vi "teleop_v4.vi"() -> ()   [LabVIEW 2012, in "MainProject.lvrbt"]
uses:
  MainProject.lvrbt
  <vilib>/NXT/Hardware/Plugins/Tetrix 180 deg Servo/Tetrix180ServoAddress.ctl
  <vilib>/NXT/Hardware/Plugins/Tetrix DC Motor/TetrixDCMotorAddress.ctl
  <vilib>/NXT/HiTechnic/HiTechnic Controls/HiTechnic Port.ctl
  <vilib>/NXT/Block Support/NXT_InputPort.ctl
  <vilib>/NXT/Hardware/Plugins/Tetrix Continuous Servo/TetrixContinuousServoAddress.ctl
  Drivers/AutoDriverControl.ctl
  <vilib>/NXT/Dual Mode Library/Advanced/NXTFlag_Get_Integer.vi
  <vilib>/NXT/NXTIO Xnodes/NXTIONodeSubVIs/TETRIX IO Stop DC Motors.vi
  <vilib>/NXT/NXTIO Xnodes/NXTIONodeSubVIs/TETRIX IO Move DC Motors.vi
  <vilib>/NXT/Dual Mode Library/Sound/Tone.vi
  <vilib>/NXT/NXTIO Xnodes/NXTIONodeSubVIs/TETRIX IO Move Servos.vi
  <vilib>/NXT/Dual Mode Library/Advanced/NXTFlag_Assign_integer.vi
  <vilib>/NXT/NXTIO Xnodes/NXTIONodeSubVIs/TETRIX IO Move Continuous Servos.vi
  <vilib>/NXT/NXTIO Xnodes/NXTIONodeSubVIs/TETRIX IO Stop Continuous Servos.vi
  <vilib>/FTC/FTC Calculate Drive Power - Tank.vi
  <vilib>/NXT/NXTIO Xnodes/NXTIONodeSubVIs/TETRIX IO Check Battery.vi
  <vilib>/NXT/Subs/LVHSConnector.ctl
  <vilib>/NXT/NXTIO Xnodes/AddressXNode/NXTIOAddress.xnode
  <vilib>/NXT/NXTIO Xnodes/NXTIOXNode/NXTIO.xnode
  <vilib>/NXT/LegoClasses/BrickReference/BrickReference.lvclass
panel:
  out "Drive Power":i8=75 min=-100 max=100
  # "This VI was generated based on your configuration in the Remote Control Editor. You may modify the code as needed for your robot. To test this program for an FTC match, return to the Remote Control Editor, select the \"Run Program\" tab, and choose \"Teleop\"."
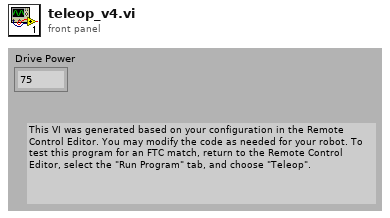
[diagram p1: front panel]
types:
  T1 = typedef "Tetrix180ServoAddress.ctl" = i16
  T2 = cluster{"Tetrix180Servo":T1, "Tetrix180Servo":T1, "Tetrix180Servo":T1}
  T3 = typedef "LVHSConnector.ctl" = refnum<class "BrickReference.lvclass">
  T4 = typedef "TetrixDCMotorAddress.ctl" = i16
  T5 = cluster{"TetrixDCMotor":T4, "TetrixDCMotor 2":T4}
  T6 = typedef "AutoDriverControl.ctl" = enum16{"Init", "Forward", "Reverse", "Left", "Right", "Brake"}
  T7 = typedef "FTC ControllerState.ctl" = cluster{"Left X":i8, "Left Y":i8, "Right X":i8, "Right Y":i8, "Button Encoding 9-12":u8, "Button Encoding 1-8":u8, "POV":T8}
  T8 = typedef "FTC POVState.ctl" = i8
  T9 = typedef "FTC ButtonEventType.ctl" = enum16{"Pressed", "Released"}
  T10 = cluster{"Button ID":enum16{"None", "Button 1", "Button 2", "Button 3", "Button 4", "Button 5", "Button 6", "Button 7", "Button 8", "Button 9", "Button 10", "Button 11", "Button 12", "POV Up", "POV Up Right", "POV Right", "POV Down Right", "POV Down", "POV Down Left", "POV Left", "POV Up Left"}, "Event Type":T9}[]
  T11 = enum16{"None", "Button 1", "Button 2", "Button 3", "Button 4", "Button 5", "Button 6", "Button 7", "Button 8", "Button 9", "Button 10", "Button 11", "Button 12", "POV Up", "POV Up Right", "POV Right", "POV Down Right", "POV Down", "POV Down Left", "POV Left", "POV Up Left"}
  T12 = typedef "TetrixContinuousServoAddress.ctl" = i16
  T13 = typedef "HiTechnic Port.ctl" = cluster{"Port":T14, "MUX Port":u8}
  T14 = typedef "NXT_InputPort.ctl" = u8
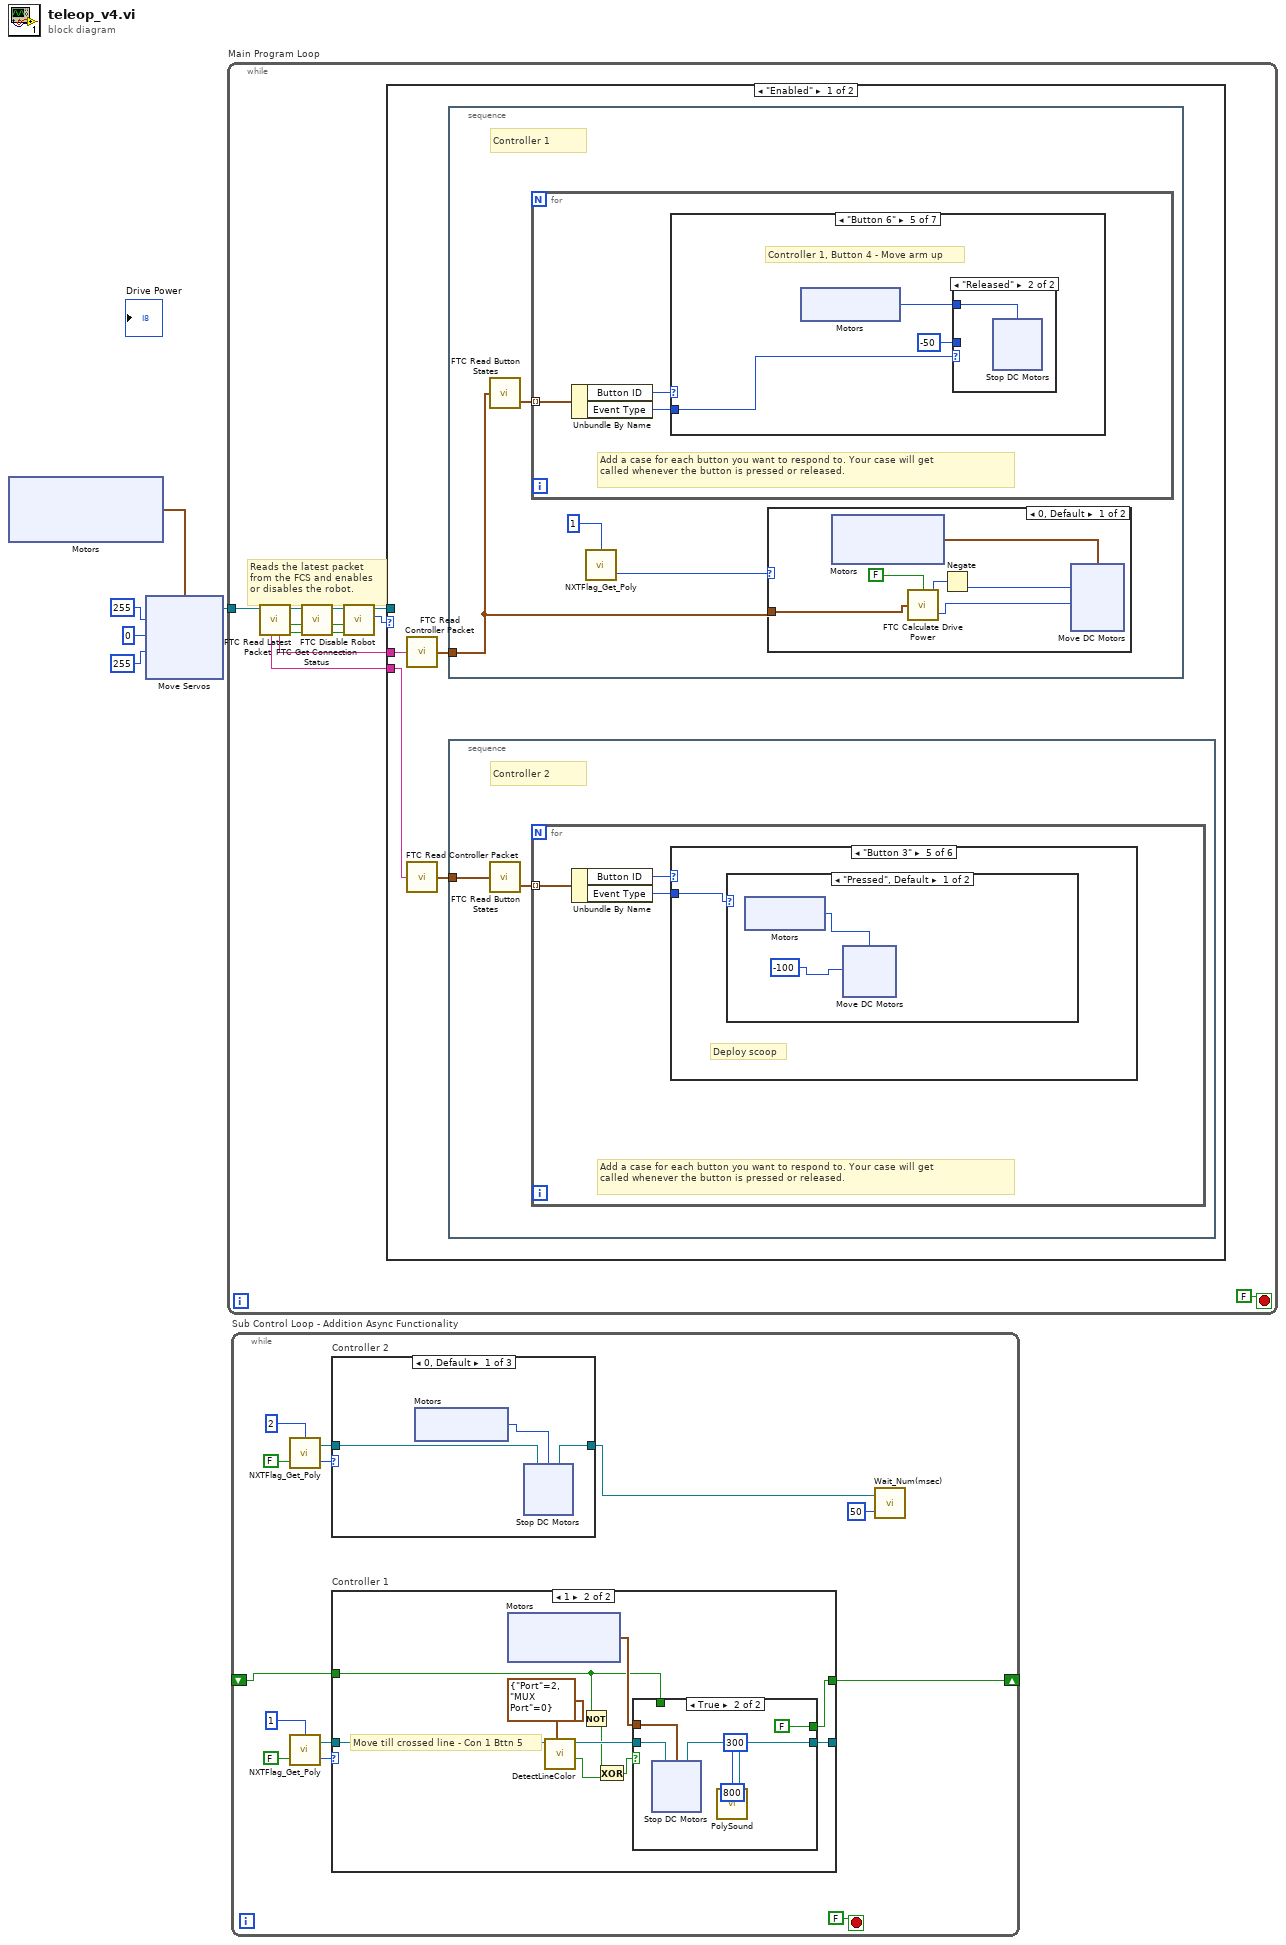
[diagram p0: block diagram]
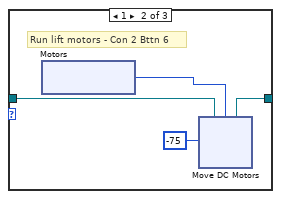
[diagram p2: hidden frame]
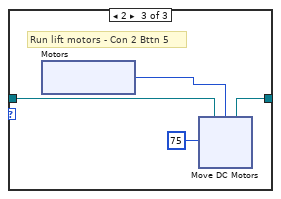
[diagram p3: hidden frame]
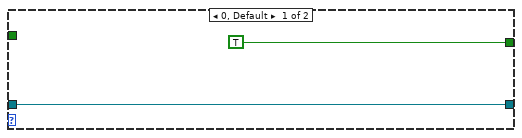
[diagram p4: hidden frame]
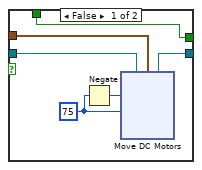
[diagram p5: hidden frame]
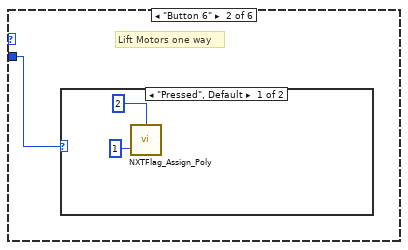
[diagram p7: hidden frame]
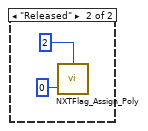
[diagram p8: hidden frame]
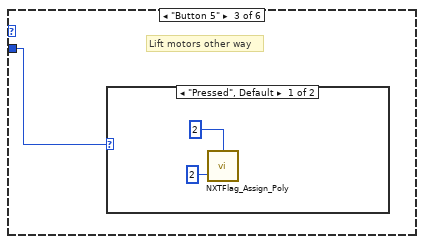
[diagram p9: hidden frame]
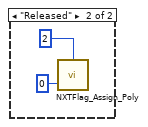
[diagram p10: hidden frame]
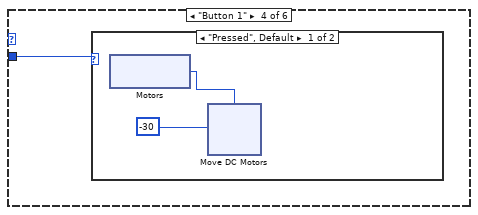
[diagram p11: hidden frame]
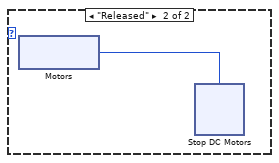
[diagram p12: hidden frame]
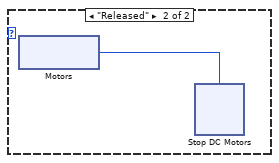
[diagram p13: hidden frame]
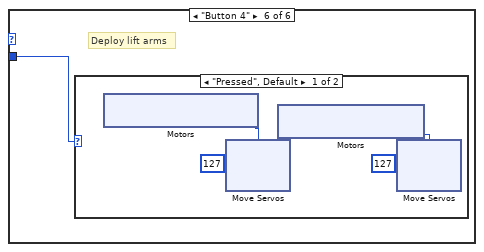
[diagram p14: hidden frame]
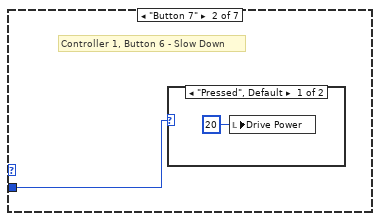
[diagram p18: hidden frame]
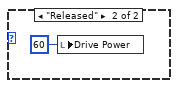
[diagram p19: hidden frame]
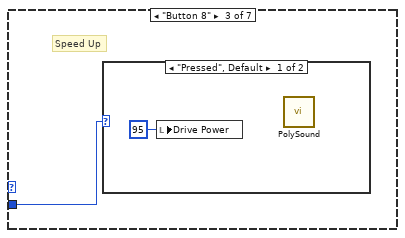
[diagram p20: hidden frame]
diagram:
  n1 = xnode "Motors"() -> ("Motor"=w4:T2)
  n2 = xnode "Move Servos"("Position 2"=u8 0, "Position 1"=u8 255, "Servos"=w4, "Position 3"=u8 255) -> ("NXT"=w5:T3)  [unwired: 1 in]
  n3 = while "Main Program Loop" {
    tunnel: w5 -> [w6]
    stop <- FALSE stop-if-true
    # "Reads the latest packet\nfrom the FCS and enables\nor disables the robot."
    n4 = call <vilib>:"FTC Read Latest Packet.vi"("NXT"=w6) -> ("Packet Received?"=w14:bool, "Stopped?"=w11:bool, "NXT"=w13:T3, "Controller 1"=w16:string, "Controller 2"=w15:string)  [unwired: 5 in, 1 out]
    n5 = call <vilib>:"FTC Get Connection Status.vi"("Packet Received?"=w14, "Stopped?"=w11, "NXT"=w13) -> ("Online?"=w8:bool, "Stopped?"=w9:bool, "NXT"=w10:T3)  [unwired: 5 in]
    n6 = call <vilib>:"FTC Disable Robot.vi"("Online?"=w8, "Stopped?"=w9, "NXT"=w10) -> ("Enabled?"=w12:enum16{"Disabled", "Enabled"}, "NXT"=w7:T3)  [unwired: 3 in]
    n7 = case "disableCase" shown="\"Enabled\"" w12 {
      tunnel: w16 -> [w21 _]
      tunnel: w15 -> [w20 _]
      tunnel: w7 -> [_ w207]
      frame "Enabled" {
        n8 = call <vilib>:"FTC Read Controller Packet.vi"("Packet"=w21) -> ("Controller State"=w19:T7)  [unwired: 4 in]
        n9 = call <vilib>:"FTC Read Controller Packet.vi"("Packet"=w20) -> ("Controller State"=w18:T7)  [unwired: 4 in]
        n10 = stacked-sequence "controller1Actions" {
          tunnel: w19 -> [w94]
          frame #0 {
            # "Controller 1"
            n11 = call <vilib>:"FTC Read Button States.vi"("Controller State"=w94) -> ("Button Events"=w97:T10)  [unwired: 2 in, 1 out]
            n12 = for "buttonAction" {
              tunnel: w97 -> [w115] mode=indexing
              # "Add a case for each button you want to respond to. Your case will get \ncalled whenever the button is pressed or released."
              n13 = Unbundle By Name(w115) -> ("Button ID"=w117:T11, "Event Type"=w116:T9)
              n14 = case "EventCase1" shown="\"Button 6\"" w117 {
                tunnel: w116 -> [_ w118 w121 w124 w134 w153 w174]
                frame Default {
                  # "No Action"
                }
                frame "Button 7" {
                  # "Controller 1, Button 6 - Slow Down"
                  n15 = case shown="\"Pressed\", Default" w118 {
                    frame "Pressed", Default {
                      n16 = local write "Drive Power"(i8 20 ("Drive Power")) -> ()
                    }
                    frame "Released" {
                      n17 = local write "Drive Power"(i8 60 ("Drive Power")) -> ()
                    }
                  }
                }
                frame "Button 8" {
                  # "Speed Up"
                  n18 = case shown="\"Pressed\", Default" w121 {
                    frame "Pressed", Default {
                      n19 = local write "Drive Power"(i8 95 ("Drive Power")) -> ()
                      n20 = call-poly <vilib>:"PolySound.vi"() -> ()  [unwired: 4 in, 1 out]
                    }
                    frame "Released" {
                      n21 = local write "Drive Power"(i8 60 ("Drive Power")) -> ()
                    }
                  }
                }
                frame "Button 2" {
                  # "Drive forward till hit line"
                  n22 = case shown="\"Released\"" w124 {
                    frame "Pressed", Default {
                      n23 = call-poly <vilib>:"NXTFlag_Assign_Poly.vi"("Flag Value"=1, "NXT Flag Number"=i8 1) -> ()  [unwired: 2 in, 1 out]
                    }
                    frame "Released" {
                      n24 = call-poly <vilib>:"NXTFlag_Assign_Poly.vi"("Flag Value"=0, "NXT Flag Number"=i8 1) -> ("NXT"=w128:T3)  [unwired: 2 in]
                      n25 = xnode "Motors"() -> ("Motor"=w130:cluster{"TetrixDCMotor":T4, "TetrixDCMotor":T4})
                      n26 = call "AutoDriver.vi"("NXT In"=w128, "Motors"=w130, "Direction"=AutoDriverControl."Brake", "Time (1 sec)"=sgl 0.0001) -> ()  [unwired: 4 in, 1 out]
                    }
                  }
                }
                frame "Button 6" {
                  # "Controller 1, Button 4 - Move arm up"
                  n27 = xnode "Motors"() -> ("Motor"=w135:T4)
                  n28 = case shown="\"Released\"" w134 {
                    tunnel: -50 ("Power (75)") -> [w139 _]
                    tunnel: w135 -> [w138 w147]
                    frame "Pressed", Default {
                      n29 = xnode "Move DC Motors"("Power/Speed 1"=w139, "Motors"=w138) -> ()  [unwired: 1 in, 1 out]
                    }
                    frame "Released" {
                      n30 = xnode "Stop DC Motors"("Motors"=w147) -> ()  [unwired: 1 in, 1 out]
                    }
                  }
                }
                frame "Button 1" {
                  # "Open Block Door Servo"
                  n31 = case shown="\"Pressed\", Default" w153 {
                    frame "Pressed", Default {
                      n32 = xnode "Motors"() -> ("Motor"=w155:T1)
                      n33 = xnode "Move Servos"("Position 1"=u8 10, "Servos"=w155) -> ()  [unwired: 1 in, 1 out]
                    }
                    frame "Released" {
                      n34 = xnode "Motors"() -> ("Motor"=w165:T1)
                      n35 = xnode "Move Servos"("Position 1"=u8 255, "Servos"=w165) -> ()  [unwired: 1 in, 1 out]
                    }
                  }
                }
                frame "Button 5" {
                  # "Controller 1, Button 2 - Move arm down"
                  n36 = xnode "Motors"() -> ("Motor"=w175:T4)
                  n37 = case shown="\"Pressed\", Default" w174 {
                    tunnel: 50 ("Power (75)") -> [w179 _]
                    tunnel: w175 -> [w178 w187]
                    frame "Pressed", Default {
                      n38 = xnode "Move DC Motors"("Power/Speed 1"=w179, "Motors"=w178) -> ()  [unwired: 1 in, 1 out]
                    }
                    frame "Released" {
                      n39 = xnode "Stop DC Motors"("Motors"=w187) -> ()  [unwired: 1 in, 1 out]
                    }
                  }
                }
              }
            }
            n40 = call-poly <vilib>:"NXTFlag_Get_Poly.vi"("NXT Flag Number"=1) -> ("Flag Value"=w95:i32)  [unwired: 2 in, 1 out]
            n41 = case shown="0, Default" w95 {
              tunnel: w94 -> [w98 _]
              frame 0, Default {
                n42 = xnode "Motors"() -> ("Motor"=w102:cluster{"TetrixDCMotor":T4, "TetrixDCMotor":T4})
                n43 = call-poly <vilib>:"FTC Calculate Drive Power.vi"("Reverse"=FALSE, "Controller State"=w98) -> ("Right Motor Power"=w100:i8, "Left Motor Power"=w101:i8)  [unwired: 2 in]
                n44 = Negate(x=w101) -> (-x=w99:i8)
                n45 = xnode "Move DC Motors"("Power/Speed 2"=w100, "Power/Speed 1"=w99, "Motors"=w102) -> ()  [unwired: 1 in, 1 out]
              }
              frame 1 {
              }
            }
          }
        }
        n46 = stacked-sequence "controller2Actions" {
          tunnel: w18 -> [w22]
          frame #0 {
            # "Controller 2"
            n47 = call <vilib>:"FTC Read Button States.vi"("Controller State"=w22) -> ("Button Events"=w23:T10)  [unwired: 2 in, 1 out]
            n48 = for "buttonAction" {
              tunnel: w23 -> [w24] mode=indexing
              # "Add a case for each button you want to respond to. Your case will get \ncalled whenever the button is pressed or released."
              n49 = Unbundle By Name(w24) -> ("Button ID"=w26:T11, "Event Type"=w25:T9)
              n50 = case "EventCase2" shown="\"Button 3\"" w26 {
                tunnel: w25 -> [_ w27 w32 w37 w55 w73]
                frame Default {
                  # "No Action"
                }
                frame "Button 6" {
                  # "Lift Motors one way"
                  n51 = case shown="\"Pressed\", Default" w27 {
                    frame "Pressed", Default {
                      n52 = call-poly <vilib>:"NXTFlag_Assign_Poly.vi"("Flag Value"=1, "NXT Flag Number"=i8 2) -> ()  [unwired: 2 in, 1 out]
                    }
                    frame "Released" {
                      n53 = call-poly <vilib>:"NXTFlag_Assign_Poly.vi"("Flag Value"=0, "NXT Flag Number"=i8 2) -> ()  [unwired: 2 in, 1 out]
                    }
                  }
                }
                frame "Button 5" {
                  # "Lift motors other way"
                  n54 = case shown="\"Pressed\", Default" w32 {
                    frame "Pressed", Default {
                      n55 = call-poly <vilib>:"NXTFlag_Assign_Poly.vi"("Flag Value"=2, "NXT Flag Number"=i8 2) -> ()  [unwired: 2 in, 1 out]
                    }
                    frame "Released" {
                      n56 = call-poly <vilib>:"NXTFlag_Assign_Poly.vi"("Flag Value"=0, "NXT Flag Number"=i8 2) -> ()  [unwired: 2 in, 1 out]
                    }
                  }
                }
                frame "Button 1" {
                  n57 = case shown="\"Pressed\", Default" w37 {
                    frame "Pressed", Default {
                      n58 = xnode "Motors"() -> ("Motor"=w39:T12)
                      n59 = xnode "Move DC Motors"("Power/Speed 1"=i8 -30, "Motors"=w39) -> ()  [unwired: 1 in, 1 out]
                    }
                    frame "Released" {
                      n60 = xnode "Motors"() -> ("Motor"=w48:T12)
                      n61 = xnode "Stop DC Motors"("Motors"=w48) -> ()  [unwired: 1 in, 1 out]
                    }
                  }
                }
                frame "Button 3" {
                  # "Deploy scoop"
                  n62 = case shown="\"Pressed\", Default" w55 {
                    frame "Pressed", Default {
                      n63 = xnode "Motors"() -> ("Motor"=w57:T12)
                      n64 = xnode "Move DC Motors"("Power/Speed 1"=i8 -100, "Motors"=w57) -> ()  [unwired: 1 in, 1 out]
                    }
                    frame "Released" {
                      n65 = xnode "Motors"() -> ("Motor"=w66:T12)
                      n66 = xnode "Stop DC Motors"("Motors"=w66) -> ()  [unwired: 1 in, 1 out]
                    }
                  }
                }
                frame "Button 4" {
                  # "Deploy lift arms"
                  n67 = case shown="\"Pressed\", Default" w73 {
                    frame "Pressed", Default {
                      n68 = xnode "Motors"() -> ("Motor"=w77:T1)
                      n69 = xnode "Move Servos"("Position 1"=u8 127, "Servos"=w77) -> ()  [unwired: 1 in, 1 out]
                      n70 = xnode "Motors"() -> ("Motor"=w75:T1)
                      n71 = xnode "Move Servos"("Position 1"=u8 127, "Servos"=w75) -> ()  [unwired: 1 in, 1 out]
                    }
                    frame "Released" {
                    }
                  }
                }
              }
            }
          }
        }
      }
      frame "Disabled" {
        w195 = 0 ("Flag Value")
        # "If the robot is disabled, read the battery voltages and stop all motors."
        n72 = xnode ("Motors")() -> ("Motor"=w206:T4)
        n73 = xnode ("Check Battery")("Motors"=w206, "NXT"=w207) -> ("Voltage 1"=w205:sgl, "NXT"=w204:T3)
        n74 = xnode "Motors"() -> ("Motor"=w203:cluster{"TetrixDCMotor":T4, "TetrixDCMotor":T4})
        n75 = call <vilib>:"MCT DisplayVoltage.vi"("Motor Voltage"=w205, "NXT"=w204) -> ("NXT"=w202:T3)  [unwired: 9 in]
        n76 = xnode "Motors"() -> ("Motor"=w201:T4)
        n77 = xnode "Move DC Motors"("Motors"=w203, "NXT"=w202) -> ("NXT"=w200:T3)
        n78 = xnode "Stop DC Motors"("Motors"=w201, "NXT"=w200) -> ("NXT"=w199:T3)
        n79 = call-poly <vilib>:"NXTFlag_Assign_Poly.vi"("Flag Value"=w195, "NXT"=w199, "NXT Flag Number"=i8 1) -> ("NXT"=w197:T3)  [unwired: 1 in]
        n80 = call-poly <vilib>:"NXTFlag_Assign_Poly.vi"("Flag Value"=w195, "NXT"=w197, "NXT Flag Number"=i8 2) -> ("NXT"=w193:T3)  [unwired: 1 in]
        n81 = xnode "Motors"() -> ("Motor"=w194:T1)
        n82 = xnode "Move Servos"("Servos"=w194, "NXT"=w193) -> ()  [unwired: 1 in, 1 out]
      }
    }
  }
  n83 = while "Sub Control Loop - Addition Async Functionality" {
    shift-right: [w239] -> _
    shift-left: _ -> [w238]
    stop <- FALSE stop-if-true
    n84 = call-poly <vilib>:"NXTFlag_Get_Poly.vi"("Clear if Found"=FALSE, "NXT Flag Number"=2) -> ("Flag Value"=w240:i32, "NXT"=w241:T3)  [unwired: 1 in]
    n85 = call-poly <vilib>:"NXTFlag_Get_Poly.vi"("Clear if Found"=FALSE, "NXT Flag Number"=1) -> ("Flag Value"=w247:i32, "NXT"=w244:T3)  [unwired: 1 in]
    n86 = case "Controller 2" shown="0, Default" w240 {
      tunnel: w241 -> [w250 w259 w271]
      tunnel: [w249 w258 w270] -> w237
      frame 0, Default {
        n87 = xnode "Motors"() -> ("Motor"=w251:T4)
        n88 = xnode "Stop DC Motors"("Motors"=w251, "NXT"=w250) -> ("NXT"=w249:T3)
      }
      frame 1 {
        # "Run lift motors - Con 2 Bttn 6"
        n89 = xnode "Motors"() -> ("Motor"=w260:T4)
        n90 = xnode "Move DC Motors"("Power/Speed 1"=i8 -75, "Motors"=w260, "NXT"=w259) -> ("NXT"=w258:T3)
      }
      frame 2 {
        # "Run lift motors - Con 2 Bttn 5"
        n91 = xnode "Motors"() -> ("Motor"=w272:T4)
        n92 = xnode "Move DC Motors"("Power/Speed 1"=i8 75, "Motors"=w272, "NXT"=w271) -> ("NXT"=w270:T3)
      }
    }
    n93 = case "Controller 1" shown="1" w247 {
      tunnel: w244 -> [w283 w291]
      tunnel: [w283 w289] -> _
      tunnel: [TRUE w288] -> w239
      tunnel: w238 -> [_ w286]
      frame 0, Default {
      }
      frame 1 {
        # "Move till crossed line - Con 1 Bttn 5"
        n94 = xnode "Motors"() -> ("Motor"=w292:cluster{"TetrixDCMotor":T4, "TetrixDCMotor":T4})
        n95 = call "DetectLineColor.vi"("Port/MUX"=T13 {"Port"=2, "MUX Port"=0}, "NXT In"=w291) -> ("Detected Line?"=w287:bool, "NXT Out"=w290:T3)  [unwired: 7 in, 1 out]
        n96 = Not(x=w286) -> (.not. x?=w284:bool)
        n97 = Exclusive Or(1:w287, 2:w284) -> (0:w285:bool)
        n98 = case shown="True" w285 {
          tunnel: w292 -> [w300 w316]
          tunnel: w290 -> [w298 w315]
          tunnel: [w297 w314] -> w289
          tunnel: w286 -> [w295 _]
          tunnel: [w295 FALSE] -> w288
          frame False {
            w299 = i8 75 ("Power/Speed 1")
            n99 = Negate(x=w299) -> (-x=w296:i8)
            n100 = xnode "Move DC Motors"("Power/Speed 2"=w299, "Power/Speed 1"=w296, "Motors"=w300, "NXT"=w298) -> ("NXT"=w297:T3)
          }
          frame True {
            n101 = xnode "Stop DC Motors"("Motors"=w316, "NXT"=w315) -> ("NXT"=w314:T3)
            n102 = call-poly <vilib>:"PolySound.vi"("Duration (500 ms)"=u16 800, "NXT"=w314, "Tone (440 Hz)"=u16 300) -> ()  [unwired: 1 in, 1 out]
          }
        }
      }
    }
    n103 = call <vilib>:"Wait_Num(msec).vi"("Time (100 msec)"=u32 50, "NXT"=w237) -> ()  [unwired: 2 in, 1 out]
  }
